vi "Create Blank Excel File.vi"(0 "Filepath In":path, 7 "TemplatePath":path, 11 "Error In":errorcluster) -> (4 "Filepath Out":path, 8 "File Created?":bool, 15 "Error Out":errorcluster)   [LabVIEW 2013]
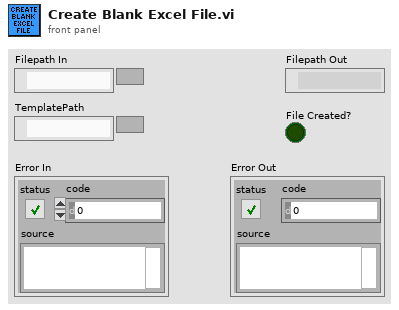
[diagram p1: front panel]
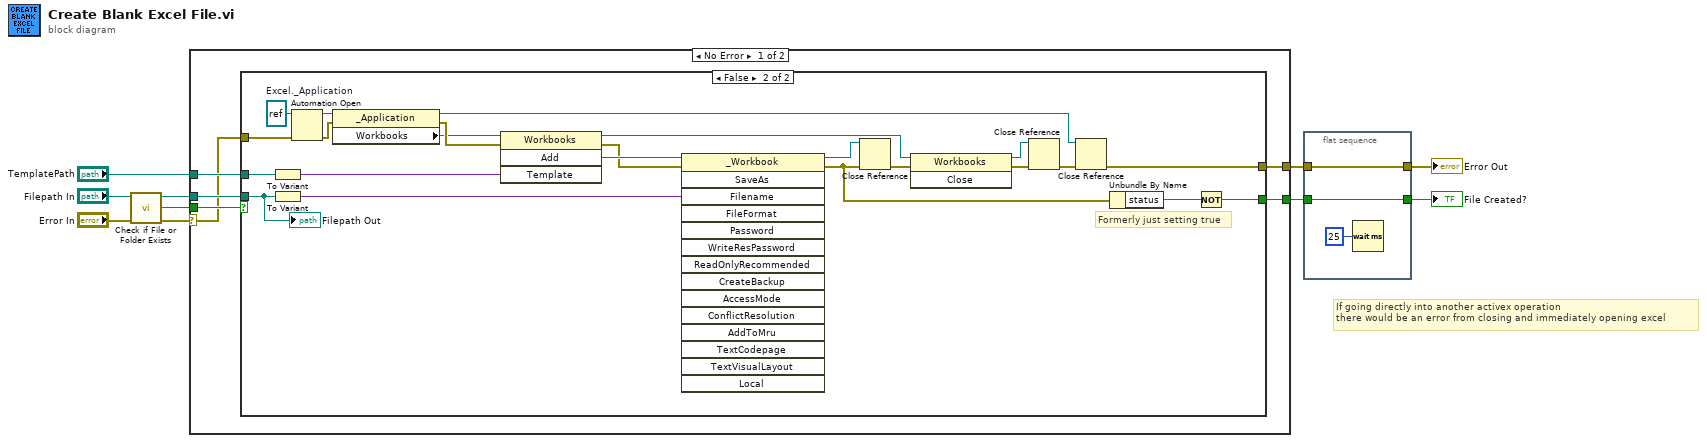
[diagram p0: block diagram]
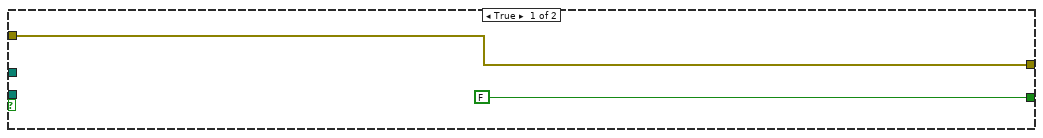
[diagram p2: hidden frame]
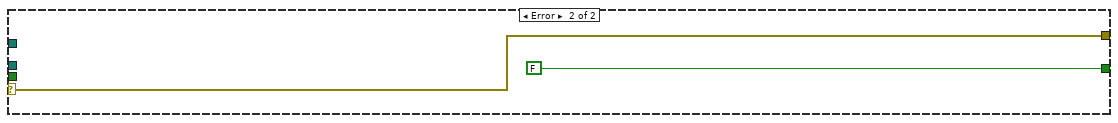
[diagram p3: hidden frame]
diagram:
  # "If going directly into another activex operation\nthere would be an error from closing and immediately opening excel"
  n1 = call <vilib>:"Check if File or Folder Exists.vi"("error in (no error)"="Error In", "path"="Filepath In") -> ("error out"=w8:errorcluster, "file or folder exists?"=w7:bool, "dup path"=w6:path)  [unwired: 7 in]
  n2 = case shown="No Error" w8 {
    selector: w8 -> [w12 w43]
    tunnel: "TemplatePath" -> [w16 _]
    tunnel: [w15 w43] -> w5
    tunnel: w7 -> [w14 _]
    tunnel: w6 -> [w13 _]
    tunnel: [w11 FALSE] -> w4
    frame No Error {
      n3 = case shown="False" w14 {
        tunnel: w16 -> [_ w30]
        tunnel: [w18 w22] -> w15
        tunnel: w13 -> [_ w32]
        tunnel: w12 -> [w18 w34]
        tunnel: [FALSE w19] -> w11
        frame True {
        }
        frame False {
          w23 = refnum<k7> refnum  # Excel._Application
          # "Formerly just setting true"
          n4 = To Variant(anything=w30) -> (Variant=w35:variant)
          n5 = To Variant(anything=w32) -> (Variant=w39:variant)
          n6 = Automation Open(error in (no error)=w34, Automation Refnum=w23) -> (Automation Refnum=w25:refnum<k7>, error out=w24:errorcluster)  [unwired: 2 in]
          n7 = property class="_Application"(reference=w25, error in=w24) -> (reference out=w37:refnum<k7>, error out=w41:errorcluster, "Workbooks"=w40:refnum<k7>)
          n8 = invoke class="Workbooks" method="Add"(reference=w40, error in=w41, "Template"=w35) -> (reference out=w31:refnum<k7>, error out=w28:errorcluster, "Add"=w29:refnum<k7>)  [unwired: 1 in, 1 out]
          n9 = invoke class="_Workbook" method="SaveAs"(reference=w29, error in=w28, "Filename"=w39) -> (reference out=w38:refnum<k7>, error out=w20:errorcluster)  [unwired: 12 in, 13 out]
          n10 = Close Reference(reference=w38, error in (no error)=w20) -> (error out=w36:errorcluster)
          n11 = invoke class="Workbooks" method="Close"(reference=w31, error in=w36) -> (reference out=w26:refnum<k7>, error out=w27:errorcluster)  [unwired: 1 in, 1 out]
          n12 = Close Reference(reference=w26, error in (no error)=w27) -> (error out=w33:errorcluster)
          n13 = Close Reference(reference=w37, error in (no error)=w33) -> (error out=w22:errorcluster)
          n14 = Unbundle By Name(w20) -> ("status"=w21:bool)
          n15 = Not(x=w21) -> (.not. x?=w19:bool)
          "Filepath Out" <- w32
        }
      }
    }
    frame Error {
    }
  }
  n16 = flat-sequence {
    tunnel: w5 -> [w46]
    tunnel: w4 -> [w45]
    tunnel: [w46] -> w3
    tunnel: [w45] -> w2
    frame #0 {
      n17 = Wait (ms)(milliseconds to wait=u32 25) -> ()  [unwired: 1 out]
    }
  }
  "Error Out" <- w3
  "File Created?" <- w2
